vi "commandStart.vi"(8 "error in (no error)":errorcluster, 10 "CommandStart in":T1, 11 "M1M3SAL in":refnum<class "M1M3SAL.lvclass">) -> (0 "error out":errorcluster, 2 "CommandStart out":T1, 3 "M1M3SAL out":refnum<class "M1M3SAL.lvclass">)   [LabVIEW 2016, in "M1M3SupportCommunicator.lvlib" / "M1M3SAL.lvclass"]
uses:
  M1M3SAL.lvclass
  DataTypes/Topics/CommandStart.ctl
  DataTypes/Topics/Parts/CommandId.ctl
  DataTypes/MessageHeader.ctl
  DataTypes/MessageTypes.ctl
  DataTypes/MessageTopics.ctl
  Common_RT_Utilities/U8ArrayBuilderAutoIndexing/U8ArrayBuilderAutoIndexing.lvclass
  M1M3SupportCommunicator.lvlib
  DataTypes/Topics/M1M3SupportTopics.lvlib
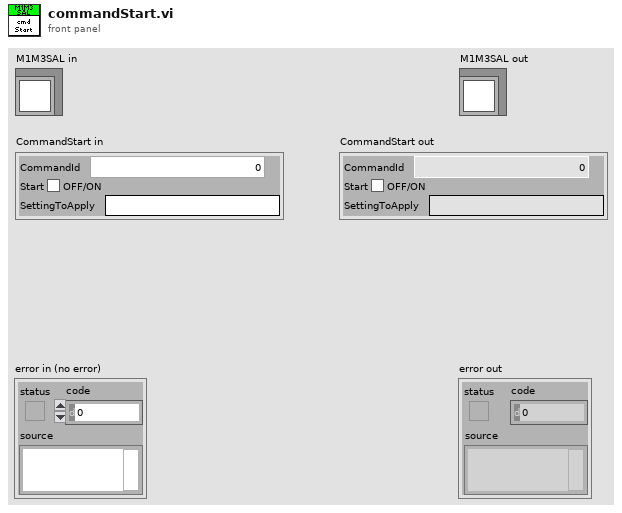
[diagram p1: front panel]
types:
  T1 = typedef "M1M3SupportTopics.lvlib/CommandStart.ctl" = cluster{"CommandId":T2, "Start":bool, "SettingToApply":string}
  T2 = typedef "M1M3SupportTopics.lvlib/CommandId.ctl" = i32
  T3 = typedef "M1M3SupportCommunicator.lvlib/MessageHeader.ctl" = cluster{"Type":T4, "Topic":T5, "Size":i32}
  T4 = typedef "M1M3SupportCommunicator.lvlib/MessageTypes.ctl" = enum8{"None", "PutSample", "GetNextSample", "LogEvent", "GetEvent", "IssueCommand", "CommandId", "WaitForCompletion", "AcceptCommand", "AckCommand"}
  T5 = typedef "M1M3SupportCommunicator.lvlib/MessageTopics.ctl" = enum8{"None", "ForceActuatorData", "MirrorForceData", "HardpointData", "AirData", "DynamicData", "FPGAData", "IMSData", "ForceActuatorStatus", "ElevationData", "HardpointStatus", "HardpointActuatorChase", "AirStatus", "ForceActuatorSafetyChecks", "ForceActuatorTest", "ActuatorBroadcastCounter", "StatusChecks", "CellChecks", "HardpointActuatorBreakaway", "RaiseMirrorComplete", "ILCCommunication", "ElevationAngleChecks", "DetailedState", "ServoLoops", "ForceActuatorInfo", "LowerMirrorComplete", "HardpointActuatorInfo", "SettingsApplied", "ErrorCode", "StartupChecks", "SummaryState", "SettingVersions", "ActuatorTestStatus", "AppliedSettingsMatchStart", "Enable", "EnterMaintenance", "Standby", "AbortLowerM1M3", "ApplyAberrationByForces", "ApplyAOSCorrectionByBendingModes", "ClearAOSCorrection", "Start", "RaiseM1M3", "TestForceActuator", "LowerM1M3", "ApplyAOSCorrectionByForces", "Disable", "ApplyAberationByBendingMode", "TestHardpoint", "ManipulateM1M3", "ClearAberration", "Exit", "TestAir", "AbortRaiseM1M3", "MoveHardpointActuators", "ExitMaintenance", "Shutdown"}
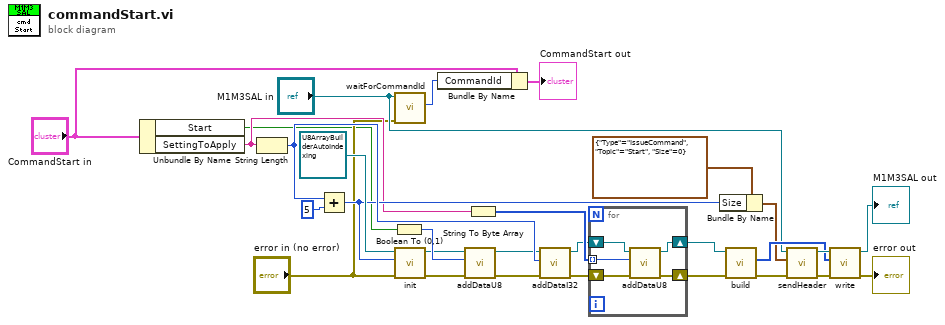
[diagram p0: block diagram]
diagram:
  n1 = Unbundle By Name("CommandStart in") -> ("Start"=w6:bool, "SettingToApply"=w20:string)
  n2 = String Length(string=w20) -> (length=w25:i32)
  n3 = Add(x=w25, y=5) -> (x+y=w21:i32)
  n4 = Boolean To (0,1)(Boolean=w6) -> (0, 1=w5:i16)
  n5 = call "waitForCommandId.vi"("error in (no error)"="error in (no error)", "M1M3SAL in"="M1M3SAL in") -> ("CommandId"=w12:T2)  [unwired: 7 in, 2 out]
  n6 = call "init.vi"("error in (no error)"="error in (no error)", "Size"=w21, "U8ArrayBuilderAutoIndexing in"=refnum<class "U8ArrayBuilderAutoIndexing.lvclass"> refnum ("RTUtilities.lvlib:U8ArrayBuilderAutoIndexing.lvclass")) -> ("error out"=w1:errorcluster, "U8ArrayBuilderAutoIndexing out"=w4:refnum<class "U8ArrayBuilderAutoIndexing.lvclass">)  [unwired: 7 in]
  n7 = Bundle By Name(cluster="CommandStart in", "CommandId"=w12) -> (→"CommandStart out":T1)
  n8 = call "addDataU8.vi"("error in (no error)"=w1, "Data"=w5, "U8ArrayBuilderAutoIndexing in"=w4) -> ("error out"=w2:errorcluster, "U8ArrayBuilderAutoIndexing out"=w3:refnum<class "U8ArrayBuilderAutoIndexing.lvclass">)  [unwired: 7 in]
  n9 = String To Byte Array(string=w20) -> (unsigned byte array=w19:u8[])
  n10 = call "addDataI32.vi"("error in (no error)"=w2, "Data"=w25, "U8ArrayBuilderAutoIndexing in"=w3) -> ("error out"=w15:errorcluster, "U8ArrayBuilderAutoIndexing out"=w18:refnum<class "U8ArrayBuilderAutoIndexing.lvclass">)  [unwired: 7 in]
  n11 = for {
    tunnel: w19 -> [w34] mode=indexing
    shift-right: [w32] -> w17
    shift-left: w18 -> [w33]
    shift-right: [w31] -> w16
    shift-left: w15 -> [w30]
    n12 = call "addDataU8.vi"("error in (no error)"=w30, "Data"=w34, "U8ArrayBuilderAutoIndexing in"=w33) -> ("error out"=w31:errorcluster, "U8ArrayBuilderAutoIndexing out"=w32:refnum<class "U8ArrayBuilderAutoIndexing.lvclass">)  [unwired: 7 in]
  }
  n13 = Bundle By Name(cluster=T3 {"Type"=enum."IssueCommand", "Topic"=enum."Start", "Size"=0} ("MessageHeader"), "Size"=w21) -> (w22:T3)
  n14 = call "build.vi"("error in (no error)"=w16, "U8ArrayBuilderAutoIndexing in"=w17) -> ("error out"=w9:errorcluster, "Array"=w27:u8[])  [unwired: 7 in, 1 out]
  n15 = call "sendHeader.vi"("error in (no error)"=w9, "MessageHeader"=w22, "M1M3SAL in"="M1M3SAL in") -> ("error out"=w26:errorcluster, "M1M3SAL out"=w28:refnum<class "M1M3SAL.lvclass">)  [unwired: 7 in]
  n16 = call "write.vi"("error in (no error)"=w26, "Data"=w27, "M1M3SAL in"=w28) -> ("error out"=→"error out":errorcluster, "M1M3SAL out"=→"M1M3SAL out":refnum<class "M1M3SAL.lvclass">)  [unwired: 7 in]
